vi "EStopMessage.vi"(8 "error in (no error)":errorcluster, 10 "MessageTxt":string, 11 "Sequence Context In":refnum<k7>) -> (0 "error out":errorcluster)   [LabVIEW 2021]
uses:
  <vilib>/addons/TestStand/_TSUtility.llb/TestStand - Start Modal Dialog (Sequence Context).vi
  <vilib>/addons/TestStand/_TSUtility.llb/TestStand - Set Property Value (Boolean).vi
  <vilib>/addons/TestStand/_TSUtility.llb/TestStand - End Modal Dialog (Sequence Context).vi
panel:
  out "MssgText":string
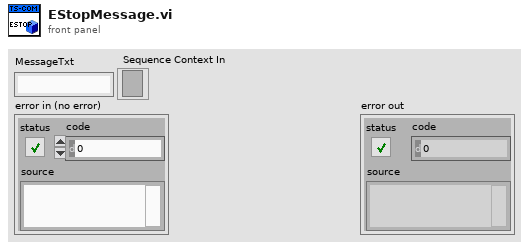
[diagram p1: front panel]
types:
  T1 = typedef "imagedata.ctl" = cluster{"image type":i32, "image depth":i32, "image":u8[], "mask":u8[], "colors":u32[], "Rectangle":cluster{"left":i16, "top":i16, "right":i16, "bottom":i16}}
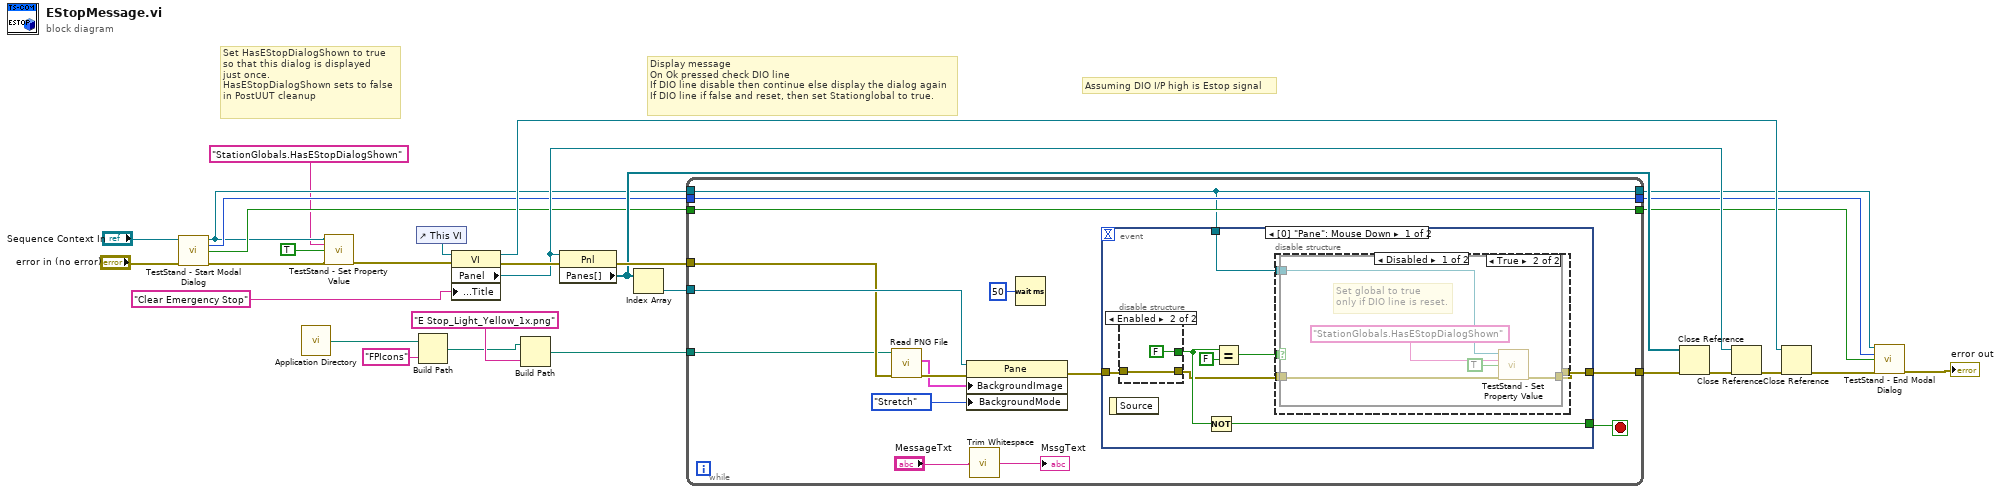
[diagram p0: block diagram]
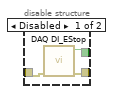
[diagram p4: hidden frame]
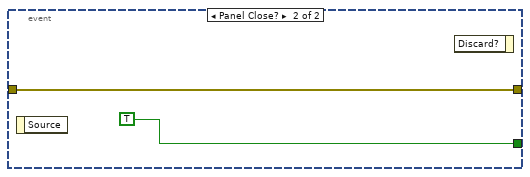
[diagram p5: hidden frame]
diagram:
  # "Set HasEStopDialogShown to true\nso that this dialog is displayed\njust once.\nHasEStopDialogShown sets to false\nin PostUUT cleanup"
  # "Assuming DIO I/P high is Estop signal"
  # "Display message\nOn Ok pressed check DIO line\nIf DIO line disable then continue else display the dialog again\nIf DIO line if false and reset, then set Stationglobal to true."
  n1 = call-poly <vilib>:"TestStand - Start Modal Dialog.vi"("Sequence Context In"="Sequence Context In", "error in (no error)"="error in (no error)") -> ("Sequence Context Out"=w2:refnum<k7>, "Modal ID"=w10:i32, "VI Originally Open"=w7:bool, "error out"=w4:errorcluster)  [unwired: 9 in, 1 out]
  n2 = call <vilib>:"Application Directory.vi"() -> ("Application Directory"=w18:path)
  n3 = call-poly <vilib>:"TestStand - Set Property Value.vi"("Sequence Context In"=w2, "Lookup String"="StationGlobals.HasEStopDialogShown", "New Value"=TRUE, "error in (no error)"=w4) -> ("error out"=w3:errorcluster)  [unwired: 10 in, 1 out]
  n4 = control-ref of="This VI"() -> (w29:refnum<vi>)
  n5 = Build Path(base path=w18, name or relative path="FPIcons") -> (appended path=w16:path)
  n6 = property class="VI"(reference=w29, error in=w3, "Front Panel.Title"="Clear Emergency Stop") -> (reference out=w24:refnum<vi>, error out=w27:errorcluster, "Panel"=w19:refnum<vi>)
  n7 = Build Path(base path=w16, name or relative path="E Stop_Light_Yellow_1x.png") -> (appended path=w15:path)
  n8 = property class="Pnl"(reference=w19, error in=w27) -> (error out=w26:errorcluster, "Panes[]"=w20:refnum<vi>[])  [unwired: 1 out]
  n9 = Index Array(array=w20) -> (element=w25:refnum<vi>)  [unwired: 1 in]
  n10 = while {
    tunnel: w26 -> [w40]
    tunnel: w25 -> [w41]
    tunnel: [w31] -> w23
    tunnel: w15 -> [w37]
    tunnel: w2 -> [w32]
    tunnel: w10 -> [w34]
    tunnel: w7 -> [w33]
    tunnel: [w32] -> w9
    tunnel: [w34] -> w8
    tunnel: [w33] -> w6
    stop <- w38 stop-if-true
    n11 = call <vilib>:"Read PNG File.vi"("error in (no error)"=w40, "path to PNG file"=w37) -> ("error out"=w43:errorcluster, "image data"=w42:T1)  [unwired: 7 in, 1 out]
    n12 = property class="Pane"(reference=w41, error in=w43, "BackgroundImage"=w42, "BackgroundMode"=enum16{"Stretch", "Center", "Tile"}."Stretch" ("Background Mode")) -> (error out=w39:errorcluster)  [unwired: 1 out]
    n13 = call <vilib>:"Trim Whitespace.vi"("string"="MessageTxt") -> ("trimmed string"=→"MssgText":string)  [unwired: 1 in]
    n14 = Wait (ms)(milliseconds to wait=u32 50) -> ()  [unwired: 1 out]
    n15 = event shown="[0] \"Pane\": Mouse Down" {
      selector: _ -> [_ _]
      dyn-events: _ -> [_ _]
      timeout: _ -> [_ _]
      tunnel: w39 -> [w53 w71]
      tunnel: [w46 w71] -> w31
      tunnel: [w52 TRUE] -> w38
      tunnel: w32 -> [w49 _]
      event Mouse Down {
        n16 = event-data() -> ()  [unwired: 1 in, 1 out]
        n17 = disable-structure shown="Enabled" {
          disable-tunnel: w53 -> [w67 w69]
          disable-tunnel: [w66 w69] -> w47
          disable-tunnel: [w65 FALSE ("DI out")] -> w51
          frame Disabled {
            n18 = call "DAQ DI_EStop.vi"("error in"=w67) -> ("error out"=w66:errorcluster, "DI out"=w65:bool)  [unwired: 9 in]
          }
          frame Enabled {
          }
        }
        n19 = Not(x=w51) -> (.not. x?=w52:bool)
        n20 = Equal?(x=w51, y=FALSE) -> (x = y?=w48:bool)
        n21 = disable-structure shown="Disabled" {
          disable-tunnel: w49 -> [w57 _]
          disable-tunnel: w48 -> [w56 _]
          disable-tunnel: w47 -> [w55 w64]
          disable-tunnel: [w54 w64] -> w46
          frame Disabled {
            n22 = case shown="True" w56 {
              tunnel: w57 -> [_ w63]
              tunnel: w55 -> [w58 w61]
              tunnel: [w58 w60] -> w54
              frame False {
              }
              frame True {
                # "Set global to true\nonly if DIO line is reset."
                n23 = call-poly <vilib>:"TestStand - Set Property Value.vi"("Sequence Context In"=w63, "Lookup String"="StationGlobals.HasEStopDialogShown", "New Value"=TRUE, "error in (no error)"=w61) -> ("error out"=w60:errorcluster)  [unwired: 10 in, 1 out]
              }
            }
          }
          frame Enabled {
          }
        }
      }
      event Panel Close? {
        n24 = event-data() -> ()  [unwired: 1 in, 1 out]
        n25 = event-data() -> ()  [unwired: 2 in, 1 out]
      }
    }
  }
  n26 = Close Reference(reference=w20, error in (no error)=w23) -> (error out=w22:errorcluster)
  n27 = Close Reference(reference=w19, error in (no error)=w22) -> (error out=w21:errorcluster)
  n28 = Close Reference(reference=w24, error in (no error)=w21) -> (error out=w13:errorcluster)
  n29 = call-poly <vilib>:"TestStand - End Modal Dialog.vi"("Sequence Context In"=w9, "Modal ID"=w8, "VI Originally Open"=w6, "error in (no error)"=w13) -> ("error out"=→"error out":errorcluster)  [unwired: 11 in]
